vi "StartScanPos_SLM.vi"(9 "Amplititute":dbl, 10 "Step Size":dbl, 11 "Number of Steps":u8) -> (1 "Start Scan Position":dbl)   [LabVIEW 2014]
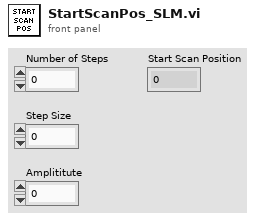
[diagram p1: front panel]
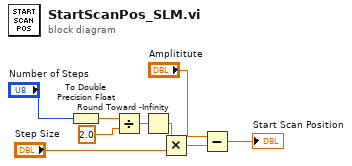
[diagram p0: block diagram]
diagram:
  n1 = To Double Precision Float(number="Number of Steps") -> (double precision float=w4:dbl)
  n2 = Divide(x=w4, y=2.0) -> (x/y=w2:dbl)
  n3 = Round Toward -Infinity(1:w2) -> (0:w1:dbl)
  n4 = Multiply(x=w1, y="Step Size") -> (x*y=w8:dbl)
  n5 = Subtract(x="Amplititute", y=w8) -> (x-y=→"Start Scan Position":dbl)
